vi "assemble.vi"(8 "error in (no error)":errorcluster, 11 "Chair in":refnum<class "Chair.lvclass">) -> (0 "error out":errorcluster, 2 "String":string="assembeld", 3 "Chair out":refnum<class "Chair.lvclass">)   [LabVIEW 2021, in "Chair.lvclass"]
uses:
  Chair.lvclass
  Furniture/Furniture.lvclass
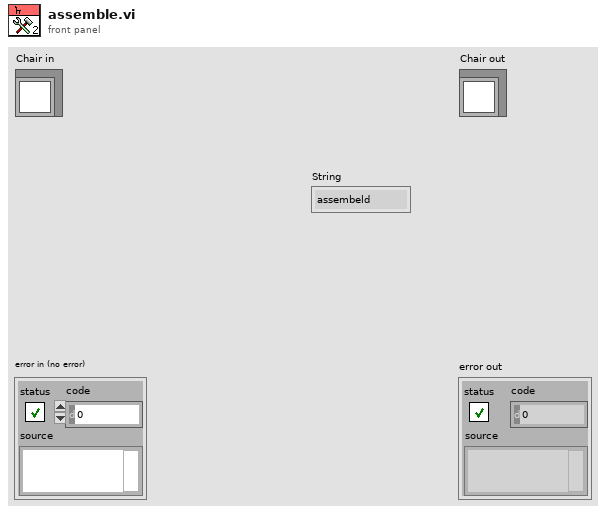
[diagram p1: front panel]
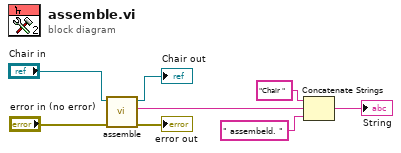
[diagram p0: block diagram]
diagram:
  n1 = call-parent "assemble.vi"("error in (no error)"="error in (no error)", "Furniture in"="Chair in") -> ("error out"=→"error out":errorcluster, "String"=w3:string, "Furniture out"=→"Chair out":refnum<class "Chair.lvclass">)  [unwired: 7 in]
  n2 = Concatenate Strings("Chair ", w3, " assembeld. ") -> (→"String":string)
